vi "add ROI element.vi"(5 "beads track":T3[](array[typedef]) {"centroid"."Y Centroid" format="%.2f"; "centroid"."X Centroid" format="%.2f"; "ROI Des out"."Contours"."Type" items=["No Selection", "Point", "Line", "Rectangle", "Oval", "Polygon", "Freehand Region", "Annulus", "Unused2", "Unused3", "Broken Line", "Freehand Line", "Rotated Rectangle"]}, 7 "beads info":T1[](array[typedef]), 9 "tracking":T3 {"centroid"."Y Centroid" format="%.2f"; "centroid"."X Centroid" format="%.2f"; "ROI Des out"."Contours"."Type" items=["No Selection", "Point", "Line", "Rectangle", "Oval", "Polygon", "Freehand Region", "Annulus", "Unused2", "Unused3", "Broken Line", "Freehand Line", "Rotated Rectangle"]}, 10 "info":T1={"data name"="", "ROI ref"=refnum, "cali ref"=refnum, "参考球？"=FALSE, "LUT"=[], "Cali array"=[], "修正次数"=2, "R_step"=0.4, "sample(quar)"=12}) -> (1 "new track":T3[](array[typedef]) {"centroid"."Y Centroid" format="%.2f"; "centroid"."X Centroid" format="%.2f"; "ROI Des out"."Contours"."Type" items=["No Selection", "Point", "Line", "Rectangle", "Oval", "Polygon", "Freehand Region", "Annulus", "Unused2", "Unused3", "Broken Line", "Freehand Line", "Rotated Rectangle"]}, 2 "new info":T1[](array[typedef]))   [LabVIEW 2017]
doc: "本VI是并行处理多个ROI信号的核心VI之一。\n本VI的功能是在ROI 引用矩阵和ROI 图像矩阵中增加一个新的元素，使得多个ROI可以整合到一起，输出到分析单元。"
uses:
  control/Bead track.ctl
  control/bead info.ctl
  <vilib>/vision/Image Controls.llb/IMAQ Image.ctl
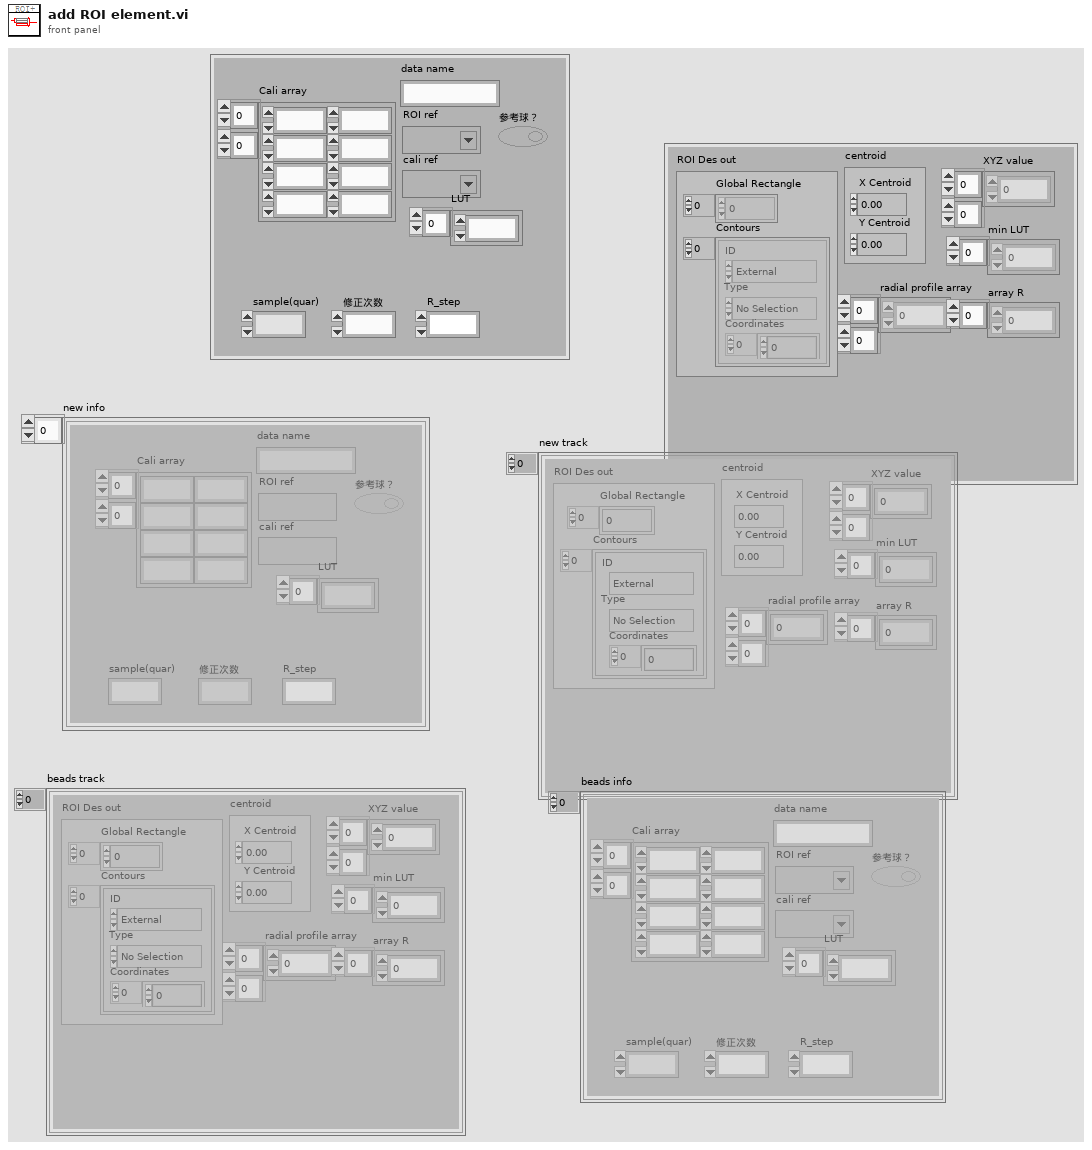
[diagram p1: front panel]
types:
  T1 = typedef "bead info.ctl" = cluster{"data name":string, "ROI ref":T2, "cali ref":T2, "参考球？":bool, "LUT":dbl[], "Cali array":dbl[][], "修正次数":i32, "R_step":dbl, "sample(quar)":i32}
  T2 = typedef "IMAQ Image.ctl" = refnum<image>
  T3 = typedef "Bead track.ctl" = cluster{"XYZ value":dbl[][], "radial profile array":dbl[][], "min LUT":dbl[], "ROI Des out":T4, "array R":dbl[], "centroid":cluster{"X Centroid":sgl, "Y Centroid":sgl}}
  T4 = typedef "ROI Descriptor" = cluster{"Global Rectangle":i32[], "Contours":cluster{"ID":enum32{"External", "Internal"}, "Type":u32, "Coordinates":i32[]}[]}
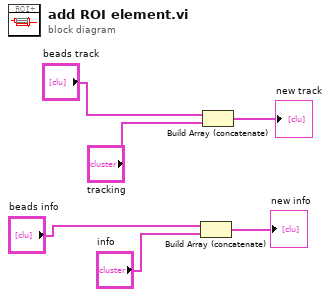
[diagram p0: block diagram]
diagram:
  n1 = Build Array (concatenate)("beads info", "info") -> (→"new info":T1[])
  n2 = Build Array (concatenate)("beads track", "tracking") -> (→"new track":T3[])
